vi "Get Valid Properties.vi"(8 "error in (no error)":errorcluster, 11 "Level in":refnum<class "Level.lvclass">) -> (0 "error out":errorcluster, 2 "Properties":string[](array[string]), 3 "Level out":refnum<class "Level.lvclass">)   [LabVIEW 2015, in "Level.lvclass"]
uses:
  Level.lvclass
  LevelUnits.ctl
panel:
  in  "Units":T1
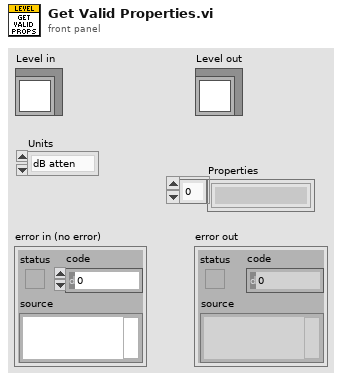
[diagram p1: front panel]
types:
  T1 = typedef "Level.lvclass/LevelUnits.ctl" = enum16{"dB atten", "dB SPL", "dB Vrms", "Volts", "dB mW", "mW", "dB HL", "dB SL"}
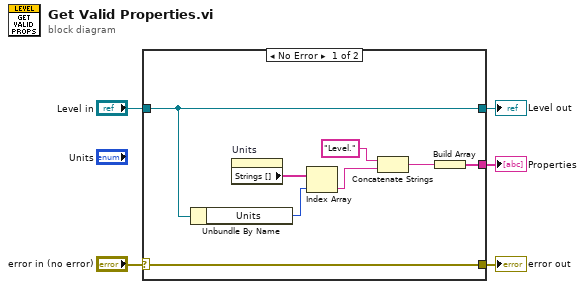
[diagram p0: block diagram]
diagram:
  n1 = case shown="No Error" "error in (no error)" {
    selector: "error in (no error)" -> [w13 w15]
    tunnel: [w13 w15] -> w4
    tunnel: [w12 w14] -> w2
    tunnel: "Level in" -> [w12 w14]
    tunnel: [w6 _] -> w1
    frame No Error {
      n2 = Unbundle By Name(w12) -> ("Units"=w10:T1)
      n3 = property on="Units" class="Enum (strict)"() -> ("Strings []"=w11:string[])  [unwired: 2 in, 2 out]
      n4 = Index Array(array=w11, index=w10) -> (element=w8:string)
      n5 = Concatenate Strings("Level.", w8) -> (w7:string)
      n6 = Build Array(w7) -> (w6:string[])
    }
    frame Error {
    }
  }
  "error out" <- w4
  "Level out" <- w2
  "Properties" <- w1
